vi "Motion_Cmd Delay.vi"(8 "error in":errorcluster, 11 "TCP Connection Refnum":refnum<k5>) -> (0 "error out":errorcluster, 3 "TCP Connection Refnum (dup)":refnum<k5>)   [LabVIEW 2010]
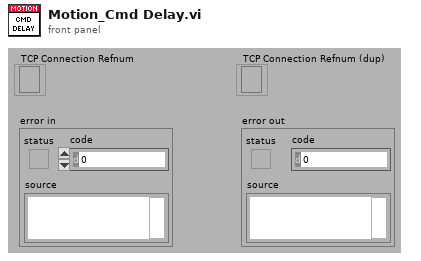
[diagram p1: front panel]
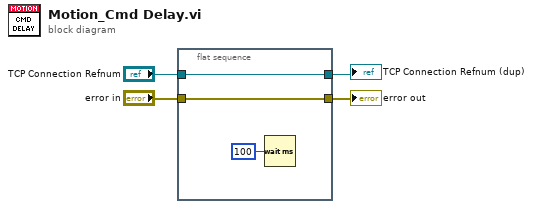
[diagram p0: block diagram]
diagram:
  n1 = flat-sequence {
    tunnel: [w7] -> w1
    tunnel: "TCP Connection Refnum" -> [w7]
    tunnel: [w6] -> w3
    tunnel: "error in" -> [w6]
    frame #0 {
      n2 = Wait (ms)(milliseconds to wait=u32 100) -> ()  [unwired: 1 out]
    }
  }
  "error out" <- w3
  "TCP Connection Refnum (dup)" <- w1
